vi "2d to boolean.vi"() -> ()   [LabVIEW 2020]
panel:
  out "initialized array":bool[][](array[boolean])
  in  "Numeric":dbl
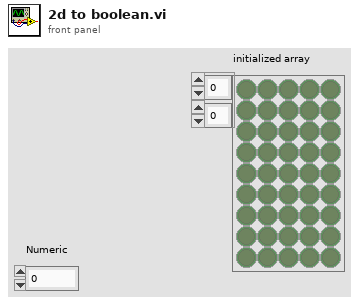
[diagram p1: front panel]
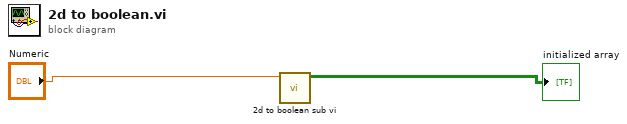
[diagram p0: block diagram]
diagram:
  n1 = call "2d to boolean sub vi.vi"("Numeric"="Numeric") -> ("initialized array"=→"initialized array":bool[][])  [unwired: 10 in]
